vi "library path.vi"() -> (3 "path":path)   [LabVIEW 2016, in "async tls dl.lvlib"]
uses:
  async tls dl.lvlib
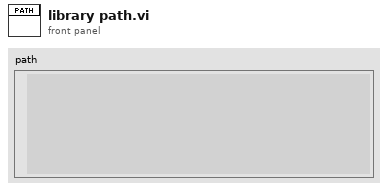
[diagram p1: front panel]
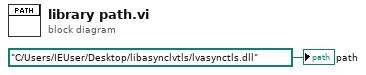
[diagram p0: block diagram]
diagram:
  "path" <- path "C:/Users/IEUser/Desktop/libasynclvtls/lvasynctls.dll" ("path")
